vi "OAT AC DC Separation (1 Channel).vi"(0 "even-angle signal":cluster{"r0":dbl, "dr":dbl, "Y":dbl[]}={"r0"=0.0, "dr"=1.0, "Y"=[]} {"r0" format="%.2p"; "dr" format="%.2p"; "Y" format="%.2f"}, 1 "even-angle channel info":T1={"channel name"="", "description"="", " channel info"={"sensor sensitivity"=1000.0, "engineering units"=1, "dB reference"=1.0, "custom label"="EU", "weighting filter"=0, "pregain"=0.0}} {"channel info"."pregain" format="%.2f"; "channel info"."weighting filter" items=["Linear", "A-weighting", "B-weighting", "C-weighting", "ITU-R 468-4", "Dolby", "CCITT", "C-message", "Wb", "Wc", "Wd", "We", "Wf", "Wh", "Wj", "Wk", "Wm", "AES17 20 kHz lowpass", "AES17 40 kHz lowpass", "AES17 20 kHz highpass", "AES17 40 kHz highpass"]; "channel info"."dB reference" format="%^.1e"; "channel info"."engineering units" items=["custom..."=0, "V"=1, "A"=21, "C"=30, "pC"=31, "s"=32, "-"=29, "Pa"=2, "N"=20, "g"=3, "m/s^2"=4, "m/s"=5, "m"=6, "mm/s"=12, "mm"=13, "micron/s"=14, "micron"=15, "in/s^2"=7, "in/s"=8, "in"=9, "mil/s"=10, "mil"=11, "rad/s^2"=16, "rad/s"=17, "rad"=18, "deg/s^2"=26, "deg/s"=27, "deg"=28, "RPM"=22, "cycle/s^2"=23, "Hz"=24, "cycle"=25, "strain"=19]; "channel info"."sensor sensitivity" format="%#_5f"}, 2 "revolution number (1)":dbl=1.0 min=0.0, 3 "position info":T5, 5 "error in (no error)":errorcluster, 8 "reset? (F)":bool) -> (12 "unit label":string, 14 "even-angle AC signal":cluster{"r0":dbl, "dr":dbl, "Y":dbl[]}={"r0"=0.0, "dr"=1.0, "Y"=[]} {"r0" format="%.2p"; "dr" format="%.2p"; "Y" format="%.2f"}, 15 "dup even-angle channel info":T1={"channel name"="", "description"="", " channel info"={"sensor sensitivity"=1000.0, "engineering units"=1, "dB reference"=1.0, "custom label"="EU", "weighting filter"=0, "pregain"=0.0}} {"channel info"."pregain" format="%.2f"; "channel info"."weighting filter" items=["Linear", "A-weighting", "B-weighting", "C-weighting", "ITU-R 468-4", "Dolby", "CCITT", "C-message", "Wb", "Wc", "Wd", "We", "Wf", "Wh", "Wj", "Wk", "Wm", "AES17 20 kHz lowpass", "AES17 40 kHz lowpass", "AES17 20 kHz highpass", "AES17 40 kHz highpass"]; "channel info"."dB reference" format="%^.1e"; "channel info"."engineering units" items=["custom..."=0, "V"=1, "A"=21, "C"=30, "pC"=31, "s"=32, "-"=29, "Pa"=2, "N"=20, "g"=3, "m/s^2"=4, "m/s"=5, "m"=6, "mm/s"=12, "mm"=13, "micron/s"=14, "micron"=15, "in/s^2"=7, "in/s"=8, "in"=9, "mil/s"=10, "mil"=11, "rad/s^2"=16, "rad/s"=17, "rad"=18, "deg/s^2"=26, "deg/s"=27, "deg"=28, "RPM"=22, "cycle/s^2"=23, "Hz"=24, "cycle"=25, "strain"=19]; "channel info"."sensor sensitivity" format="%#_5f"}, 16 "even-angle DC signal":cluster{"r0":dbl, "dr":dbl, "Y":dbl[]}={"r0"=0.0, "dr"=1.0, "Y"=[]} {"r0" format="%.2p"; "dr" format="%.2p"; "Y" format="%.2f"}, 17 "position info out":T5, 19 "error out":errorcluster)   [LabVIEW 2017, in "SoundVib_OAUtility.lvlib"]
doc: "Separates and returns the AC and DC levels of the <B>even-angle signal</B> by continuously removing the DC values from the signal. This VI calculates the DC values over the interval specified by the <B>revolution number</B>. Wire data to the <B>even-angle signal</B> input to determine the polymorphic instance to use or manually select the instance."
uses:
  <vilib>/addons/Sound and Vibration/Order Analysis/Utility/SoundVib_OAUtility.lvlib
  <vilib>/addons/_NISVFA/_Shared subVIs/Controls/svc_Resampled Channel Info.ctl
  <vilib>/addons/_NISVFA/_Shared subVIs/Controls/svc_Channel Info.ctl
  <vilib>/addons/_NISVFA/_Shared subVIs/Controls/svc_Engineering Units Text Ring.ctl
  <vilib>/addons/_NISVFA/_Shared subVIs/Controls/svc_Weighting Filter Text Ring.ctl
  <vilib>/addons/Sound and Vibration/Order Analysis/Misc/OAT Position Info.ctl
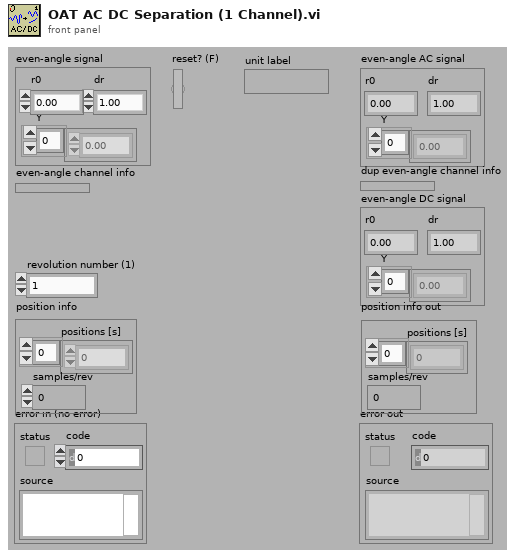
[diagram p1: front panel]
types:
  T1 = typedef "svc_Resampled Channel Info.ctl" = cluster{"channel name":string, "description":string, " channel info":T2}
  T2 = typedef "svc_Channel Info.ctl" = cluster{"sensor sensitivity":dbl, "engineering units":T3, "dB reference":dbl, "custom label":string, "weighting filter":T4, "pregain":dbl}
  T3 = typedef "svc_Engineering Units Text Ring.ctl" = u16
  T4 = typedef "svc_Weighting Filter Text Ring.ctl" = u16
  T5 = typedef "OAT Position Info.ctl" = cluster{"positions [s]":dbl[], "samples/rev":dbl}
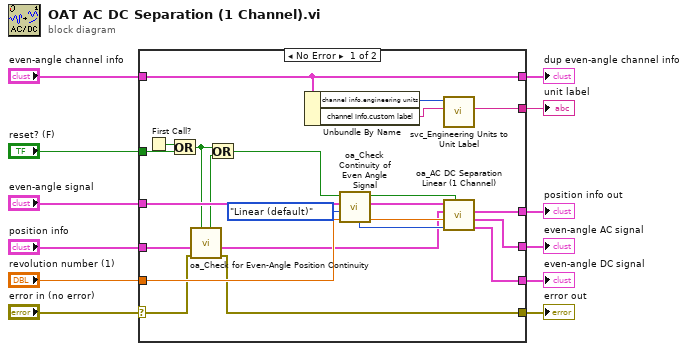
[diagram p0: block diagram]
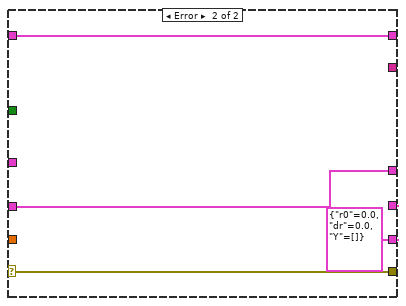
[diagram p2: hidden frame]
diagram:
  n1 = case shown="No Error" "error in (no error)" {
    selector: "error in (no error)" -> [w17 w39]
    tunnel: [w16 w39] -> w11
    tunnel: "reset? (F)" -> [w35 _]
    tunnel: "even-angle signal" -> [w33 _]
    tunnel: "even-angle channel info" -> [w24 w38]
    tunnel: [w30 w36] -> w7
    tunnel: [w29 w36] -> w6
    tunnel: "revolution number (1)" -> [w25 _]
    tunnel: [w24 w38] -> w4
    tunnel: [w15 _] -> w3
    tunnel: "position info" -> [w23 w37]
    tunnel: [w22 w37] -> w1
    frame No Error {
      n2 = First Call?() -> (First Call?: T/F=w34:bool)
      n3 = Or(x=w34, y=w35) -> (x .or. y?=w20:bool)
      n4 = call <vilib>:"oa_Check for Even-Angle Position Continuity.vi"("reset in"=w20, "error in (no error)"=w17, "even-angle position info"=w23) -> ("error out"=w16:errorcluster, "even-angle position info dup"=w21:T5, "position not continuous"=w18:bool)  [unwired: 6 in]
      n5 = Or(x=w20, y=w18) -> (x .or. y?=w19:bool)
      n6 = Unbundle By Name(w24) -> ("channel info.engineering units"=w14:T3, "channel info.custom label"=w13:string)
      n7 = call <vilib>:"oa_Check Continuity of Even Angle Signal.vi"("averaging revolution (1)"=w25, "averaging type"=enum16{"Linear (default)", "Exponential", "Mix"}."Linear (default)", "even angle signal"=w33, "reset?(F)"=w19) -> ("dul averaging revolution"=w27:dbl, "dul even angle signal"=w31:cluster{"r0":dbl, "dr":dbl, "Y":dbl[]}, "reset out"=w32:bool, "points/rev"=w28:u32)  [unwired: 3 in, 1 out]
      n8 = call <vilib>:"svc_Engineering Units to Unit Label.vi"("custom label"=w13, "engineering units"=w14) -> ("unit label"=w15:string)  [unwired: 8 in, 1 out]
      n9 = call <vilib>:"oa_AC DC Separation Linear (1 Channel).vi"("reset? (F)"=w32, "points/rev"=w28, "averaging revolution (1)"=w27, "position info"=w21, "even angle signal"=w31) -> ("DC even angle signal"=w29:cluster{"r0":dbl, "dr":dbl, "Y":dbl[]}, "AC even angle signal"=w30:cluster{"r0":dbl, "dr":dbl, "Y":dbl[]}, "position info out"=w22:T5)  [unwired: 3 in, 1 out]
    }
    frame Error {
      w36 = cluster{"r0":dbl, "dr":dbl, "Y":dbl[]} {"r0"=0.0, "dr"=0.0, "Y"=[]} ("dul even angle signal")
    }
  }
  "error out" <- w11
  "even-angle DC signal" <- w6
  "even-angle AC signal" <- w7
  "position info out" <- w1
  "unit label" <- w3
  "dup even-angle channel info" <- w4
